vi "Orion PDU Set Outlets On or Off.vi"(7 "On?":bool, 8 "error in (no error)":errorcluster, 9 "State":bool[](array[boolean]), 10 "addr":string, 11 "client handle":T1) -> (0 "error out":errorcluster, 1 "command":string, 2 "addr dup":string, 3 "client handle out":T1)   [LabVIEW 2022 SP3, in "Orion PDU.lvclass"]
uses:
  Orion PDU.lvclass
  <vilib>/httpClient/ClientHandle.ctl
  <vilib>/httpClient/POSTBuffer.vi
  <vilib>/httpClient/LabVIEWHTTPClient.lvlib
panel:
  out "body":string
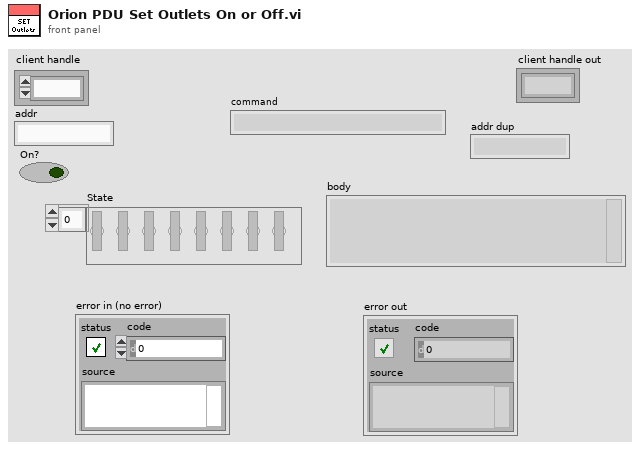
[diagram p1: front panel]
types:
  T1 = typedef "LabVIEWHTTPClient.lvlib/ClientHandle.ctl" = refnum<k1>
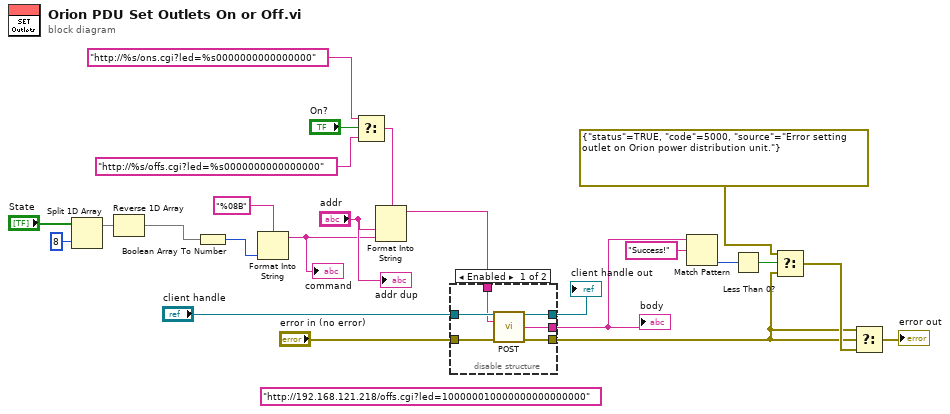
[diagram p0: block diagram]
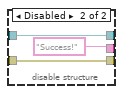
[diagram p2: hidden frame]
diagram:
  (unwired) "http://192.168.121.218/offs.cgi?led=100000010000000000000000"
  n1 = Split 1D Array(array="State", index=8) -> (first subarray=w19:bool[])  [unwired: 1 out]
  n2 = Reverse 1D Array(array=w19) -> (reversed array=w2:bool[])
  n3 = Boolean Array To Number(Boolean array=w2) -> (number=w23:u32)
  n4 = Format Into String(format string="%08B", w23) -> (resulting string=w1:string)  [unwired: 2 in, 1 out]
  "command" <- w1
  n5 = Select(t="http://%s/ons.cgi?led=%s0000000000000000", s="On?", f="http://%s/offs.cgi?led=%s0000000000000000") -> (s? t:f=w7:string)
  n6 = Format Into String(format string=w7, "addr", w1) -> (resulting string=w18:string)  [unwired: 2 in, 1 out]
  n7 = disable-structure shown="Enabled" {
    disable-tunnel: "client handle" -> [w30 w33]
    disable-tunnel: w18 -> [w29 _]
    disable-tunnel: "error in (no error)" -> [w28 w32]
    disable-tunnel: [w27 "Success!" ("regular expression")] -> w16
    disable-tunnel: [w26 w32] -> w9
    disable-tunnel: [w25 w33] -> w4
    frame Enabled {
      n8 = call-poly <vilib>:"POST.vi"("client handle"=w30, "url"=w29, "error in (no error)"=w28) -> ("client handle out"=w25:T1, "body"=w27:string, "error out"=w26:errorcluster)  [unwired: 9 in, 1 out]
    }
    frame Disabled {
    }
  }
  "body" <- w16
  "client handle out" <- w4
  n9 = Match Pattern(string=w16, regular expression="Success!") -> (offset past match=w14:i32)  [unwired: 1 in, 3 out]
  n10 = Less Than 0?(x=w14) -> (x < 0?=w13:bool)
  n11 = Select(t=errorcluster {"status"=TRUE, "code"=5000, "source"="Error setting outlet on Orion power distribution unit."} ("error out"), s=w13, f=w9) -> (s? t:f=w11:errorcluster)
  n12 = Select(t=w9, s=w9, f=w11) -> (s? t:f=→"error out":errorcluster)
  "addr dup" <- "addr"
